vi "Click to Image Coordinates.vi"(8 "error in":errorcluster, 10 "Display Reference":refnum<vi>, 11 "Coords":T1) -> (0 "error out":errorcluster, 3 "Image Coordinates":refnum<class "Vec3d.lvclass">)   [LabVIEW 2023]
uses:
  <vilib>/Utility/miscctls.llb/LVPoint32TypeDef.ctl
  Vec3d Class/Vec3d.lvclass
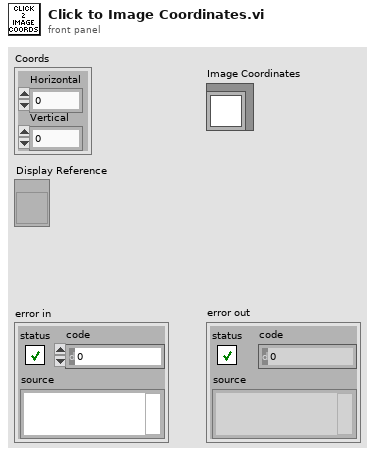
[diagram p1: front panel]
types:
  T1 = typedef "LVPoint32TypeDef.ctl" = cluster{"Horizontal":i32, "Vertical":i32}
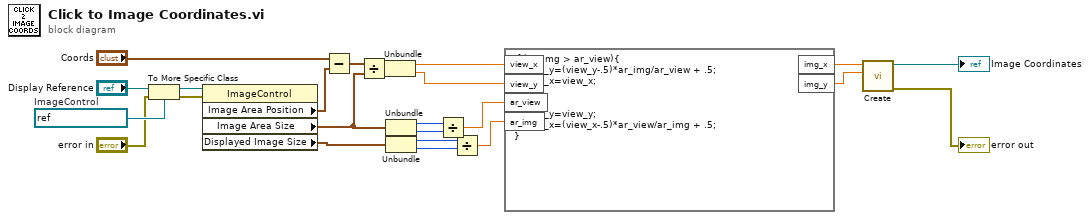
[diagram p0: block diagram]
diagram:
  w23 = refnum<vi> refnum  # ImageControl
  n1 = To More Specific Class(target class=w23, reference="Display Reference", error in="error in") -> (specific class reference=w19:refnum<vi>, error out=w14:errorcluster)
  n2 = property class="ImageControl"(reference=w19, error in=w14) -> ("Image Area Position"=w21:cluster{"Left":i32, "Top":i32}, "Image Area Size"=w10:cluster{"Width":u32, "Height":u32}, "Displayed Image Size"=w9:cluster{"Width":u32, "Height":u32})  [unwired: 2 out]
  n3 = Subtract(x="Coords", y=w21) -> (x-y=w20:T1)
  n4 = Divide(x=w20, y=w10) -> (x/y=w17:cluster{dbl, dbl})
  n5 = Unbundle(w17) -> (w12:dbl, w11:dbl)
  n6 = Unbundle(w10) -> ("Width"=w8:u32, "Height"=w7:u32)
  n7 = Unbundle(w9) -> ("Width"=w6:u32, "Height"=w5:u32)
  n8 = Divide(x=w8, y=w7) -> (x/y=w4:dbl)
  n9 = Divide(x=w6, y=w5) -> (x/y=w3:dbl)
  n10 = formula code="if (ar_img > ar_view){\n    img_y=(view_y-.5)*ar_img/ar_view + .5;\n    img_x=view_x;\n}\nelse{\n    img_y=view_y;\n    img_x=(view_x-.5)*ar_view/ar_img + .5;\n}"("view_x"=w12, "view_y"=w11, "ar_view"=w4, "ar_img"=w3) -> ("img_x"=w2:dbl, "img_y"=w1:dbl)
  n11 = call "Create.vi"("Y"=w1, "X"=w2) -> ("error out"=→"error out":errorcluster, "Vec3d Class out"=→"Image Coordinates":refnum<class "Vec3d.lvclass">)  [unwired: 8 in]
